vi "path list.vi"() -> ()   [LabVIEW 2018]
panel:
  in  "path list":path[](array[path])
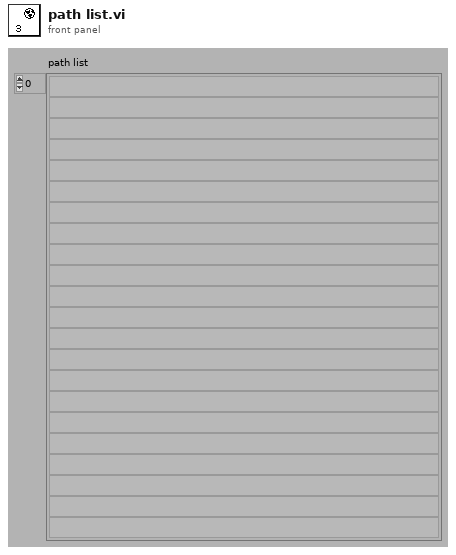
[diagram p1: front panel]
diagram:
